vi "Get_APC_Limit_Power_dBm.vi"(8 "error in (no error)":errorcluster, 11 ".NET Reference in":refnum<k24>) -> (0 "error out":errorcluster, 1 "maxpow":dbl, 2 "minpow":dbl, 3 "Reference out":refnum<k24>)   [LabVIEW 2017]
uses:
  C:/Users/Ssantec_Test/Documents/Installment_DLL_Sample_Labview_20211104/DLL/x86/InstrumentDLL.dll
  DLL/x86/InstrumentDLL.dll
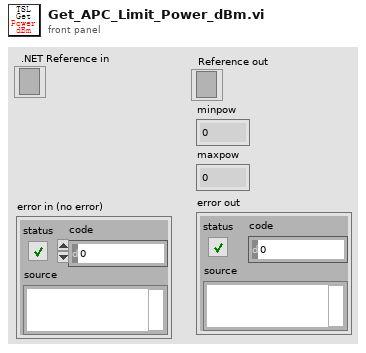
[diagram p1: front panel]
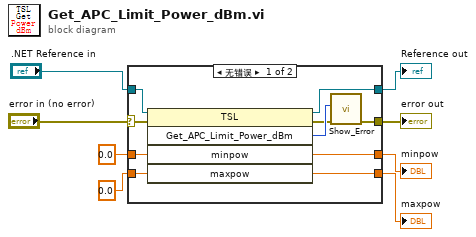
[diagram p0: block diagram]
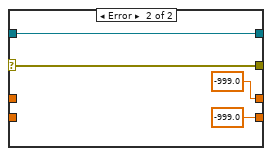
[diagram p2: hidden frame]
diagram:
  n1 = case shown="无错误" "error in (no error)" {
    selector: "error in (no error)" -> [w9 w22]
    tunnel: ".NET Reference in" -> [w18 w21]
    tunnel: [w17 w21] -> w7
    tunnel: [w10 w22] -> w6
    tunnel: [w16 -999.0 ("minpow")] -> w5
    tunnel: [w15 -999.0 ("maxpow")] -> w4
    tunnel: 0.0 ("minpow") -> [w14 _]
    tunnel: 0.0 ("maxpow") -> [w13 _]
    frame No Error {
      n2 = invoke on="调用节点" class="TSL" method="Get_APC_Limit_Power_dBm"(reference=w18, error in=w9, "minpow"=w14, "maxpow"=w13) -> (reference out=w17:refnum<k24>, error out=w11:errorcluster, "Get_APC_Limit_Power_dBm"=w12:i32, "minpow"=w16:dbl, "maxpow"=w15:dbl)  [unwired: 1 in]
      n3 = call "Show_Error.vi"("error in (no error)"=w11, "Error"=w12) -> ("error out"=w10:errorcluster)  [unwired: 9 in]
    }
    frame Error {
    }
  }
  "Reference out" <- w7
  "error out" <- w6
  "minpow" <- w5
  "maxpow" <- w4
